vi "get_description.vi"(8 "error in (no error)":errorcluster, 11 "CondimentDecorator in":refnum<class "CondimentDecorator.lvclass">) -> (0 "error out":errorcluster, 2 "Description":string, 3 "CondimentDecorator out":refnum<class "CondimentDecorator.lvclass">)   [LabVIEW 2021, in "CondimentDecorator.lvclass"]
uses:
  CondimentDecorator.lvclass
  Beverage/Beverage.lvclass
  CondimentDecorator.lvclass/CondimentDecorator.ctl
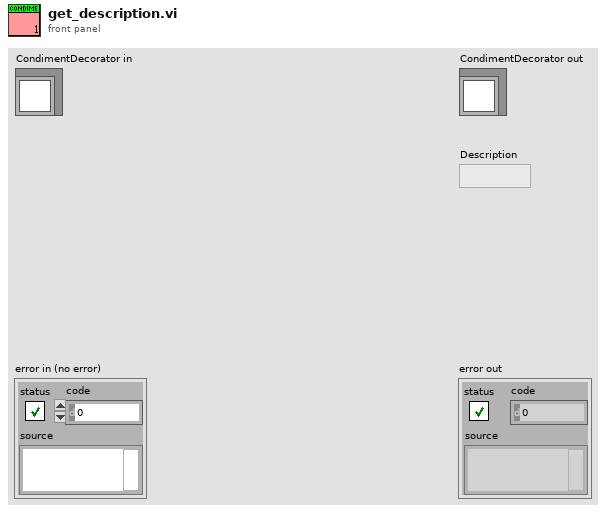
[diagram p1: front panel]
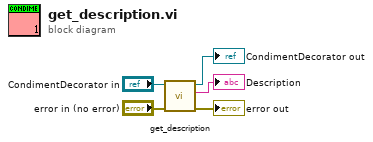
[diagram p0: block diagram]
diagram:
  n1 = call-parent "get_description.vi"("error in (no error)"="error in (no error)", "Beverage in"="CondimentDecorator in") -> ("error out"=→"error out":errorcluster, "Description"=→"Description":string, "Beverage out"=→"CondimentDecorator out":refnum<class "CondimentDecorator.lvclass">)  [unwired: 7 in]
